vi "Read TM Config.vi"(8 "error in (no error)":errorcluster) -> (0 "error out":errorcluster, 1 "Standard H20 Mass @ 60":dbl, 2 "Cal Temp Coefficient":dbl, 3 "Config Path ourt":path, 4 "TempCorrection":dbl, 5 "Report Path":path)   [LabVIEW 2018]
uses:
  <vilib>/Utility/config.llb/Read Key (Double).vi
  <vilib>/Utility/config.llb/Read Key (Path).vi
  <vilib>/Utility/config.llb/NI_LVConfig.lvlib
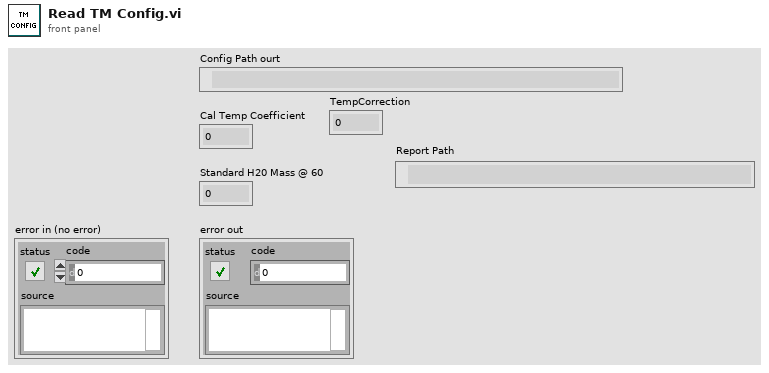
[diagram p1: front panel]
types:
  T1 = typedef "NI_LVConfig.lvlib/Config Data RefNum.ctl" = refnum<k1>
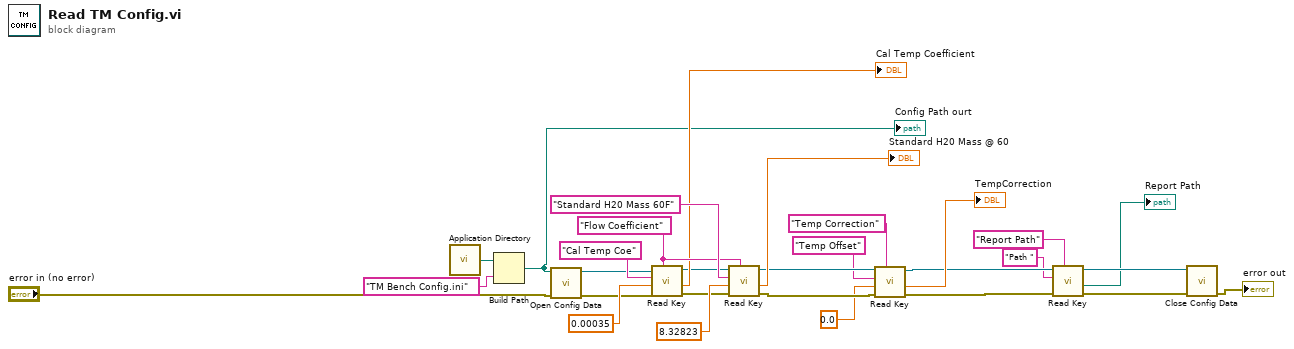
[diagram p0: block diagram]
diagram:
  w25 = "Flow Coefficient" ("section")
  n1 = call <vilib>:"Application Directory.vi"() -> ("Application Directory"=w15:path)
  n2 = Build Path(base path=w15, name or relative path="TM Bench Config.ini") -> (appended path=w17:path)
  "Config Path ourt" <- w17
  n3 = call <vilib>:"Open Config Data.vi"("error in (no error)"="error in (no error)", "configuration file path"=w17) -> ("error out"=w19:errorcluster, "refnum"=w18:T1)  [unwired: 7 in, 1 out]
  n4 = call-poly <vilib>:"Read Key.vi"("section"=w25, "error in (no error)"=w19, "default value"=0.00035, "key"="Cal Temp Coe", "refnum"=w18) -> ("error out"=w24:errorcluster, "value"=→"Cal Temp Coefficient":dbl, "refnum out"=w22:T1)  [unwired: 3 in, 1 out]
  n5 = call-poly <vilib>:"Read Key.vi"("section"=w25, "error in (no error)"=w24, "default value"=8.32823, "key"="Standard H20 Mass 60F", "refnum"=w22) -> ("error out"=w13:errorcluster, "value"=→"Standard H20 Mass @ 60":dbl, "refnum out"=w14:T1)  [unwired: 3 in, 1 out]
  n6 = call-poly <vilib>:"Read Key.vi"("section"="Temp Correction", "error in (no error)"=w13, "default value"=0.0, "key"="Temp Offset", "refnum"=w14) -> ("error out"=w7:errorcluster, "value"=→"TempCorrection":dbl, "refnum out"=w8:T1)  [unwired: 3 in, 1 out]
  n7 = call-poly <vilib>:"Read Key.vi"("section"="Report Path", "error in (no error)"=w7, "key"="Path ", "refnum"=w8) -> ("error out"=w3:errorcluster, "value"=→"Report Path":path, "refnum out"=w6:T1)  [unwired: 4 in, 1 out]
  n8 = call <vilib>:"Close Config Data.vi"("error in (no error)"=w3, "refnum"=w6) -> ("error out"=→"error out":errorcluster)  [unwired: 8 in, 1 out]
